vi "borders and shading constant.vi"() -> (0 "borders and shading":T1={"OutsideLineStyle"=0, "OutsideColorIndex"=0, "OutsideLineWidth"=2, "BackgroundPatternColor"=4278190080} {"OutsideLineWidth" items=["wdLineWidth025pt"=2, "wdLineWidth050pt"=4, "wdLineWidth075pt"=6, "wdLineWidth100pt"=8, "wdLineWidth150pt"=12, "wdLineWidth225pt"=18, "wdLineWidth300pt"=24, "wdLineWidth450pt"=36, "wdLineWidth600pt"=48]; "OutsideLineStyle" items=["wdLineStyleNone", "wdLineStyleSingle", "wdLineStyleDot", "wdLineStyleDashSmallGap", "wdLineStyleDashLargeGap", "wdLineStyleDashDot", "wdLineStyleDashDotDot", "wdLineStyleDouble", "wdLineStyleTriple", "wdLineStyleThinThickSmallGap", "wdLineStyleThickThinSmallGap", "wdLineStyleThinThickThinSmallGap", "wdLineStyleThinThickMedGap", "wdLineStyleThickThinMedGap", "wdLineStyleThinThickThinMedGap", "wdLineStyleThinThickLargeGap", "wdLineStyleThickThinLargeGap", "wdLineStyleThinThickThinLargeGap", "wdLineStyleSingleWavy", "wdLineStyleDoubleWavy", "wdLineStyleDashDotStroked", "wdLineStyleEmboss3D", "wdLineStyleEngrave3D", "wdLineStyleOutset", "wdLineStyleInset"]})   [LabVIEW 2017, in "NI_ReportGenerationToolkit.lvlib"]
doc: "Defines the borders and shading attributes of a document."
uses:
  <vilib>/addons/_office/NI_ReportGenerationToolkit.lvlib
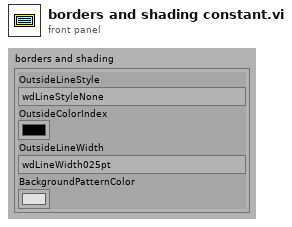
[diagram p1: front panel]
types:
  T1 = cluster{"OutsideLineStyle":i32, "OutsideColorIndex":u32, "OutsideLineWidth":i32, "BackgroundPatternColor":u32}
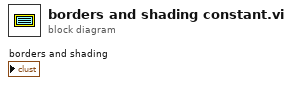
[diagram p0: block diagram]
diagram:
